vi "MGI Report Error.vi"(8 "error in":errorcluster) -> (0 "no error":errorcluster)   [LabVIEW 2020, in "MGI Error Reporter Base.lvclass"]
doc: "This reentrant VI will send a wired error or warning to the error reporter daemon. If no error reporter daemon is running or if the processing queue is full, then the error or warning is discarded.\n\nAuthored by Shawn Walpole\nsupport@mooregoodideas.com\nwww.mooregoodideas.com\n\nCopyright (c) 2013, Moore Good Ideas, Inc.\n\nAll rights reserved.\n\nRedistribution and use in source and binary forms, with or without modification, are permitted provided that the following conditions are met:\n\n * Redistributions of source code must retain the above copyright notice, this list of conditions and the following disclaimer.\n * Redistributions in binary form must reproduce the above copyright notice, this list of conditions and the following disclaimer in the documentation and/or other materials provided with the distribution.\n * Neither the name of Moore Good Ideas, Inc. nor the names of its contributors may be used to endorse or promote products derived from this software without specific prior written permission.\n\nTHIS SOFTWARE IS PROVIDED BY THE COPYRIGHT HOLDERS AND CONTRIBUTORS \"AS IS\" AND ANY EXPRESS OR IMPLIED WARRANTIES, INCLUDING, BUT NOT LIMITED TO, THE IMPLIED WARRANTIES OF MERCHANTABILITY AND FITNESS FOR A PARTICULAR PURPOSE ARE DISCLAIMED. IN NO EVENT SHALL THE COPYRIGHT OWNER OR CONTRIBUTORS BE LIABLE FOR ANY DIRECT, INDIRECT, INCIDENTAL, SPECIAL, EXEMPLARY, OR CONSEQUENTIAL DAMAGES (INCLUDING, BUT NOT LIMITED TO, PROCUREMENT OF SUBSTITUTE GOODS OR SERVICES; LOSS OF USE, DATA, OR PROFITS; OR BUSINESS INTERRUPTION) HOWEVER CAUSED AND ON ANY THEORY OF LIABILITY, WHETHER IN CONTRACT, STRICT LIABILITY, OR TORT (INCLUDING NEGLIGENCE OR OTHERWISE) ARISING IN ANY WAY OUT OF THE USE OF THIS SOFTWARE, EVEN IF ADVISED OF THE POSSIBILITY OF SUCH DAMAGE."
uses:
  <userlib>/_MGI/Error Reporter/MGI Error Reporter Base/MGI Error Reporter Base.lvclass
  <userlib>/_MGI/Error Reporter/MGI Error Reporter Base/Private/MGI Globals.vi
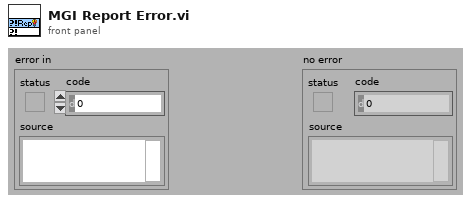
[diagram p1: front panel]
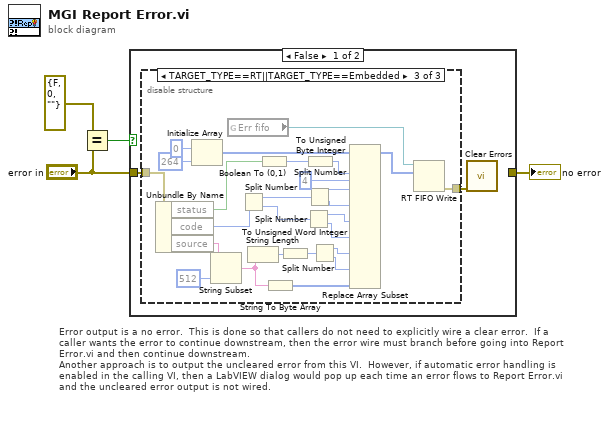
[diagram p0: block diagram]
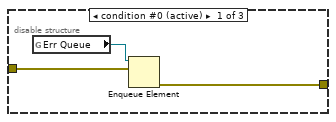
[diagram p2: hidden frame]
diagram:
  # "Error output is a no error.  This is done so that callers do not need to explicitly wire a clear error.  If a caller wants the error to continue downstream, then the error wire must branch before going into Report Error.vi and then continue downstream.\nAnother approach is to output the uncleared error from this VI.  However, if automatic error handling is enabled in the calling VI, then a LabVIEW dialog would pop up each time an error flows to Report Error.vi and the uncleared error output is not wired."
  n1 = Equal?(x=errorcluster {"status"=FALSE, "code"=0, "source"=""}, y="error in") -> (x = y?=w3:bool)
  n2 = case shown="False" w3 {
    tunnel: "error in" -> [w6 w36]
    tunnel: [_ w36] -> w2
    frame False {
      n3 = disable-structure shown="TARGET_TYPE==RT||TARGET_TYPE==Embedded" {
        disable-tunnel: w6 -> [w7 _ w15]
        disable-tunnel: [w8 _ w35] -> w5
        frame condition #0 (active) {
          n4 = global read "MGI Globals.vi" "Err Queue"() -> (w9:refnum<queue>)
          n5 = Enqueue Element(queue=w9, element=w7) -> (error out=w8:errorcluster)  [unwired: 1 in, 3 out]
        }
        frame condition #1 {
          # "Not Supported"
        }
        frame condition #2 {
          n6 = Unbundle By Name(w15) -> ("status"=w29:bool, "code"=w24:i32, "source"=w27:string)
          n7 = Initialize Array(u8 0 ("element"), 264 ("element")) -> (w31:u8[])
          n8 = String Subset(string=w27, length (rest)=512 ("length (rest)")) -> (substring=w25:string)  [unwired: 1 in]
          n9 = global read "MGI Globals.vi" "Err fifo"() -> (w34:refnum<k33>)
          n10 = Split Number(x=w24) -> (hi(x)=w19:u16, lo(x)=w18:u16)
          n11 = String Length(string=w25) -> (length=w14:i32)
          n12 = Boolean To (0,1)(Boolean=w29) -> (0, 1=w17:i16)
          n13 = String To Byte Array(string=w25) -> (unsigned byte array=w12:u8[])
          n14 = To Unsigned Word Integer(number=w14) -> (unsigned 16bit integer=w13:u16)
          n15 = Split Number(x=w18) -> (hi(x)=w21:u8, lo(x)=w20:u8)
          n16 = To Unsigned Byte Integer(number=w17) -> (unsigned 8bit integer=w16:u8)
          n17 = Split Number(x=w19) -> (hi(x)=w23:u8, lo(x)=w22:u8)
          n18 = Split Number(x=w13) -> (hi(x)=w11:u8, lo(x)=w10:u8)
          n19 = Replace Array Subset(array=w31, new element #1=w16, new element #2=w23, index #2=4 ("index"), new element #3=w22, new element #4=w21, new element #5=w20, new element #6=w11, new element #7=w10, new element #8=w12) -> (w30:u8[])  [unwired: 7 in]
          n20 = RT FIFO Write(0:w34, 1:w30) -> (11:w35:errorcluster)  [unwired: 3 in, 3 out]
        }
      }
      n21 = call <vilib>:"Clear Errors.vi"("error in (no error)"=w5) -> ()  [unwired: 1 in, 6 out]
    }
    frame True {
    }
  }
  "no error" <- w2
